vi "task3_2.vi"() -> ()   [LabVIEW 2021]
panel:
  out "data":dynamicdata(graph)
  in  "number of samples":i32=100
  in  "rate":dbl=1000.0
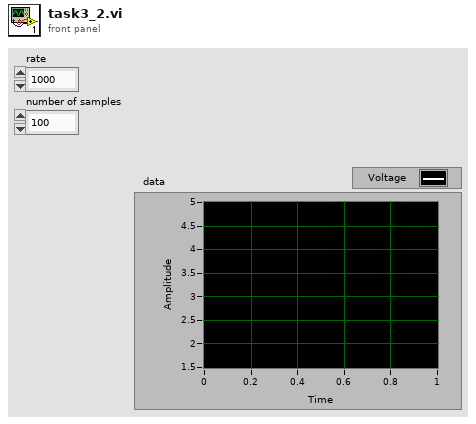
[diagram p1: front panel]
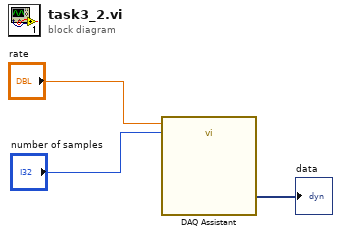
[diagram p0: block diagram]
diagram:
  n1 = call "DAQ Assistant"("rate"="rate", "number of samples"="number of samples") -> ("data"=→"data":dynamicdata)  [unwired: 15 in, 2 out]
